vi "AOD Control (host).vi"() -> ()   [LabVIEW 2009]
uses:
  <vilib>/rvi/interface/nirviOpenFPGA/nirviOpenFPGA.xnode
  <vilib>/rvi/interface/nirviReadWriteControl/nirviReadWriteControl.xnode
  <vilib>/rvi/interface/nirviMethod/nirviMethod.xnode
  <vilib>/LabVIEW Targets/FPGA/Rio/nirio_PxiTriggers.ctl
  <vilib>/rvi/interface/nirviCloseFPGA/nirviCloseFPGA.xnode
  C:/Program Files/National Instruments/LabVIEW 2009/resource/objmgr/daqmx.rc
  <vilib>/Utility/error.llb/DialogType.ctl
  <vilib>/DAQmx/write.llb/DAQmx Write (Digital Bool 1Line 1Point).vi
  <vilib>/Analysis/NI_AALBase.lvlib
  <instrlib>/niHWS/nihws.llb/niHWS Write Analog I32.vi
  <instrlib>/niHWS/nihws.llb/niHWS Open File Permissions ID.ctl
  <vilib>/DAQmx/create/channels.llb/DAQmx Create Channel (DO-Digital Output).vi
  <vilib>/DAQmx/read.llb/DAQmx Read (Raw 1D I32).vi
  <instrlib>/niHWS/nihws.llb/niHWS Write Analog I16.vi
  <vilib>/DAQmx/write.llb/DAQmx Write (Analog DBL 1Chan 1Samp).vi
  FPGA Bitfiles/AOD Control.lvproj_PXI-7954R_AOD Control (FPGA)~D2.lvbitx
  AOD Control (FPGA).vi
  AODRef.ctl
  FPGA Bitfiles/AOD Control.lvproj_PXIe-7965R_AOD Control (FPGA)~D2.lvbitx
  <vilib>/FPGA/interface/niFpgaViExecutionMode.ctl
  <vilib>/rvi/errors/niLvFpgaMergeErrorWithErrorCode.vi
  <vilib>/rvi/interface/RandomDataEmulation/nirviRandomDataDMAMethods.vi
  <vilib>/rvi/interface/common/niFpgaNodeNameForErrorReporting.ctl
  <vilib>/rvi/interface/RandomDataEmulation/niFpgaReadControlTemplate.vi
  <vilib>/rvi/interface/RandomDataEmulation/nirviRandomDataRunMethod.vi
  <vilib>/rvi/interface/RandomDataEmulation/niFpgaWriteControlTemplate.vi
  <vilib>/rvi/interface/RandomDataEmulation/nirviRandomDataClose.vi
  <vilib>/userdefined/High Color/nirio_resource_hc.ctl
panel:
  in  "Max":u32=700000
  in  "GridPoints":dbl=5.0
  in  "Power":dbl(slide) min=0.0 max=5.0 step=0.1 scale=0.0..5.0
  out "OutOfRange":bool
  out "Processing":bool
  out "Acquire":bool
  out "FPGA State":T1(ring)
  out "Host State":T2(ring)
  out "Scanning Your Mom":dbl(slide) scale=0.0..1.0
  in  "Tab Control":T3(tab)=enum."Miscellaneous"
  in  "Display Data":bool=TRUE
  in  "ClearPoints":bool
  in  "Scan Settings":T4={"XStart"=-200000000, "XEnd"=200000000, "XNum"=500, "YStart"=-200000000, "YEnd"=200000000, "YNum"=500, "ZStart"=0, "ZEnd"=0, "ZNum"=1}
  in  "Points":i32[][](array[numeric])
  in  "Stop":bool
  in  "Scan":bool
  in  "Volume Scan":bool
  in  "Abort":bool
  in  "Reset":bool
  out "Writing":bool
  in  "SaveStream":bool
  in  "SaveImage":bool
  in  "Path":path
  in  "Scans":i32=5
  in  "ImCh1":bool=TRUE
  in  "Ephys":bool
  in  "Photodiode":bool
  in  "ImCh2":bool
  in  "Throwaway (us)":i32=10
  out "PointArray":cluster{"X":i32, "Y":i32, "Z":i32}[](array[cluster])
  out "StreamInfo":T5
  in  "Downsample":i32=40
  in  "DDS SysClk":i32=100000000
  in  "FPGA Clk":i32=40000000
  in  "ImReadSize":i32=10000
  in  "AcqDivider":i32=20
  out "Acq Freq":dbl format="%#_8g"
  out "Loop Count":i32
  out "PointTime":u32
  out "PMT FIFO Space":u32
  out "ImCh Backlog":u32
  out "FPGA PMT Remaining":u32
  out "PMT Backlog":u32
  out "Command":i16
  in  "P high":u32=10
  in  "P":bool
  out "PMT Read":i32
  out "FPGA Loop Count":i32
  out "Point":cluster{"X":i32, "Y":i32, "Z":i32}
  out "TotalSamples":u32
  out "Written":cluster{"Address":u8, "Value":u32}[](array[cluster]) {"Address" format="%x"; "Value" format="%x"}
  out "PMT Array":i32[](array[numeric])
  out "ImCh Read":i32
  out "Mode":enum16{"Points", "Volume", "Idle"}(ring)
  out "FPGA VI Execution Mode":T6
  out "StackSize":cluster{"nX":u32, "nY":u32, "nZ":u32}
  out "raw out":refnum<queue>
  out "voxel queue":refnum<queue>
  out "NumChans":u32
  out "XPos":i32[](array[numeric])
  out "TRIG0":bool
  out "ExtAcqTrig":bool
  out "TriggerAcq":bool=TRUE
  out "Armed":bool
  out "Bad PMTData":bool
  out "SerialError":bool
  out "Sequencing error":bool
  out "YPos":i32[](array[numeric])
  out "ZPos":i32[](array[numeric])
  out "Point Freq":dbl
  out "SampleCount":u32
  out "AcqDivCount":u32
  out "# pending remove":i32
  out "Processed":i32
  in  "BlankTime (us)":i16=10
  out "BlankSamples":u32
  out "Throwaway Samples":dbl
  out "RepNum":i32
  out "NumReps":i32
  out "NumPoints":i32
  out "PointNum":u32
  out "LaserPowerTask":refnum<k21>
  in  "Execute":bool
  in  "Debug Mode":T7(ring)
  in  "Space":i32
  in  "decimating factor":i32=10
  in  "BaselineRate":dbl=0.01 min=0.0 max=1.0
  in  "RIO Device":T8="RIO0"
  out "ImData":i32[][](array[numeric])
  out "ImCh1 2":T9(plugin-control)
  out "ImCh2 2":T9(plugin-control)
  in  "Section":i32(c297)
  out "Waveform Chart":waveform(dbl)[](graph)
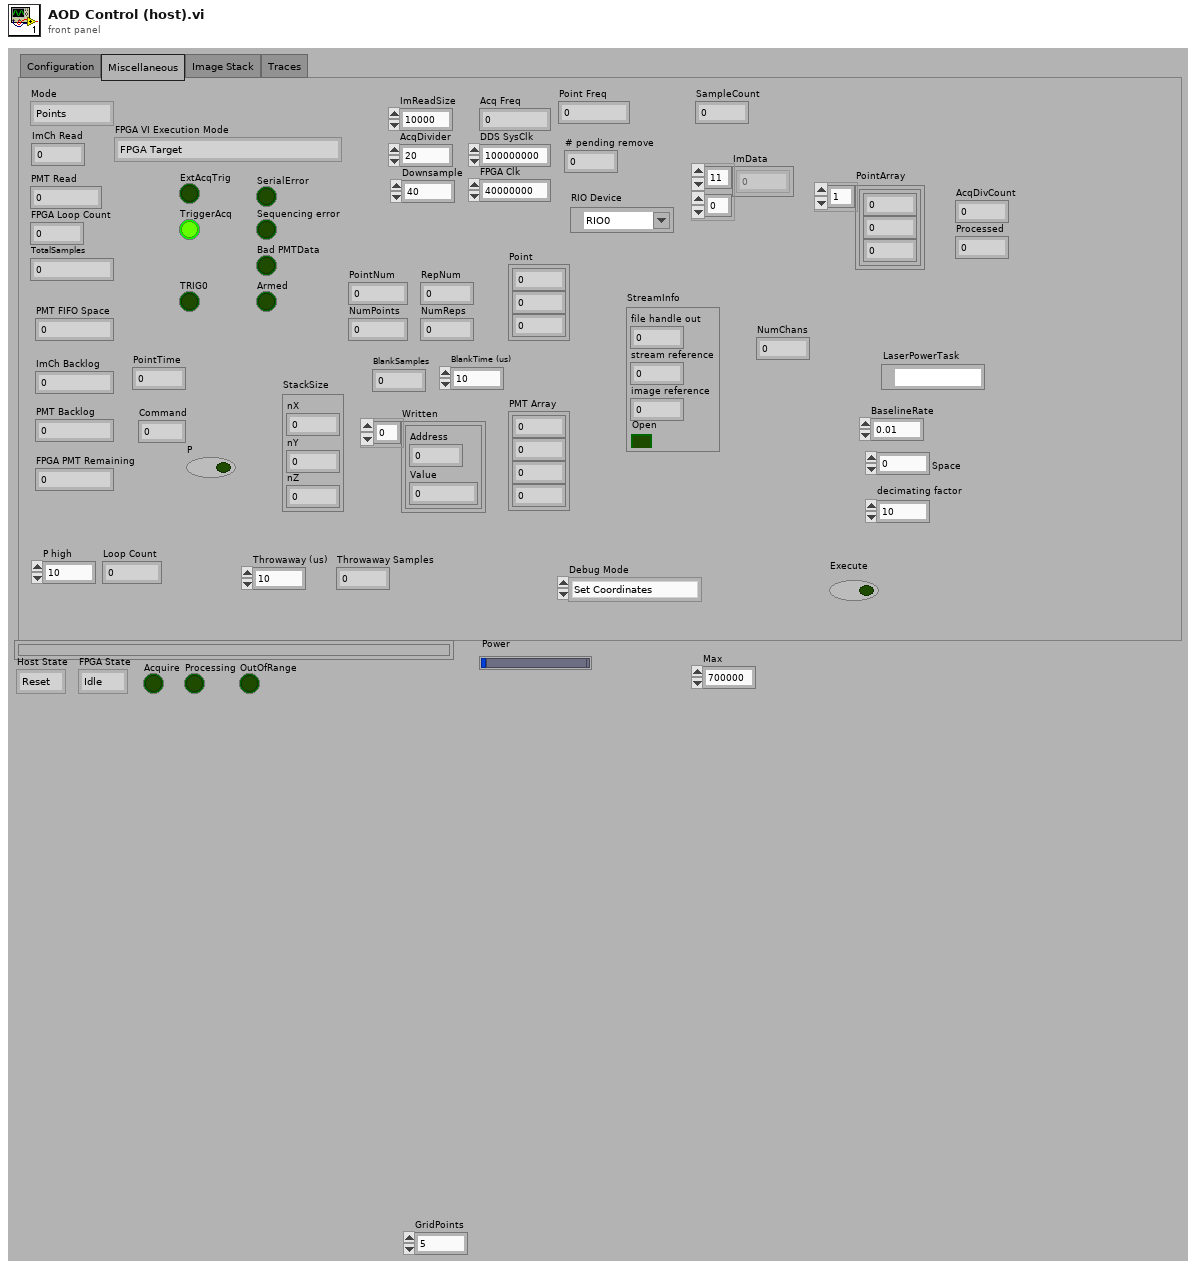
[diagram p1: front panel]
types:
  T1 = enum16{"Idle", "Write Registers", "Receive Points", "Prepare Volume", "Arm Scan", "Scan Points"}
  T2 = enum16{"Reset", "Idle", "Start Acquire", "Acquire", "End Acquire"}
  T3 = enum32{"Configuration", "Miscellaneous", "Image Stack", "Traces"}
  T4 = cluster{"XStart":i32, "XEnd":i32, "XNum":i32, "YStart":i32, "YEnd":i32, "YNum":i32, "ZStart":i32, "ZEnd":i32, "ZNum":i32}
  T5 = cluster{"file handle out":u32, "stream reference":u32, "image reference":u32, "Open":bool}
  T6 = typedef "niFpgaViExecutionMode.ctl" = enum16{"FPGA Target", "Development Computer with Simulated I/O", "Development Computer with Real I/O"}
  T7 = enum16{"Set Coordinates", "Toggle Axis", "Sweep Settings"}
  T8 = typedef "nirio_resource_hc.ctl" = tag
  T9 = typedef "IMAQ Image.ctl" = refnum<image>
  T10 = typedef "AODRef.ctl" = refnum<k20>
  T11 = typedef "nirio_PxiTriggers.ctl" = u16
  T12 = typedef "niFpgaNodeNameForErrorReporting.ctl" = enum16{"Open FPGA VI Reference", "Read/Write Control", "Invoke Method: Abort", "Invoke Method: Acknowledge IRQ", "Invoke Method: Download", "Invoke Method: FIFO.Configure", "Invoke Method: FIFO.Read", "Invoke Method: FIFO.Start", "Invoke Method: FIFO.Stop", "Invoke Method: FIFO.Write", "Invoke Method: Reset", "Invoke Method: Run", "Invoke Method: Wait on IRQ", "Close FPGA VI Reference"}
  T13 = typedef "niHWS Open File Permissions ID.ctl" = enum32{"Read Only", "Read/Write Existing", "Read/Write/Create New", "Read/Write/Create New Always"}
  T14 = typedef "Image Type" = u32
  T15 = typedef "DialogType.ctl" = u16
  T16 = cluster{"Global Rectangle":i32[], "Contours":cluster{"Contour Type":u32, "ROI Type":u32, "Points":i32[]}[]}
  T17 = cluster{"Global Rectangle":i32[], "Contours":cluster{"Contour Type":u32, "ROI Type":u32, "Points":i32[]}[]}[]
  T18 = cluster{"Contour Type":u32, "ROI Type":u32, "Points":i32[]}[]
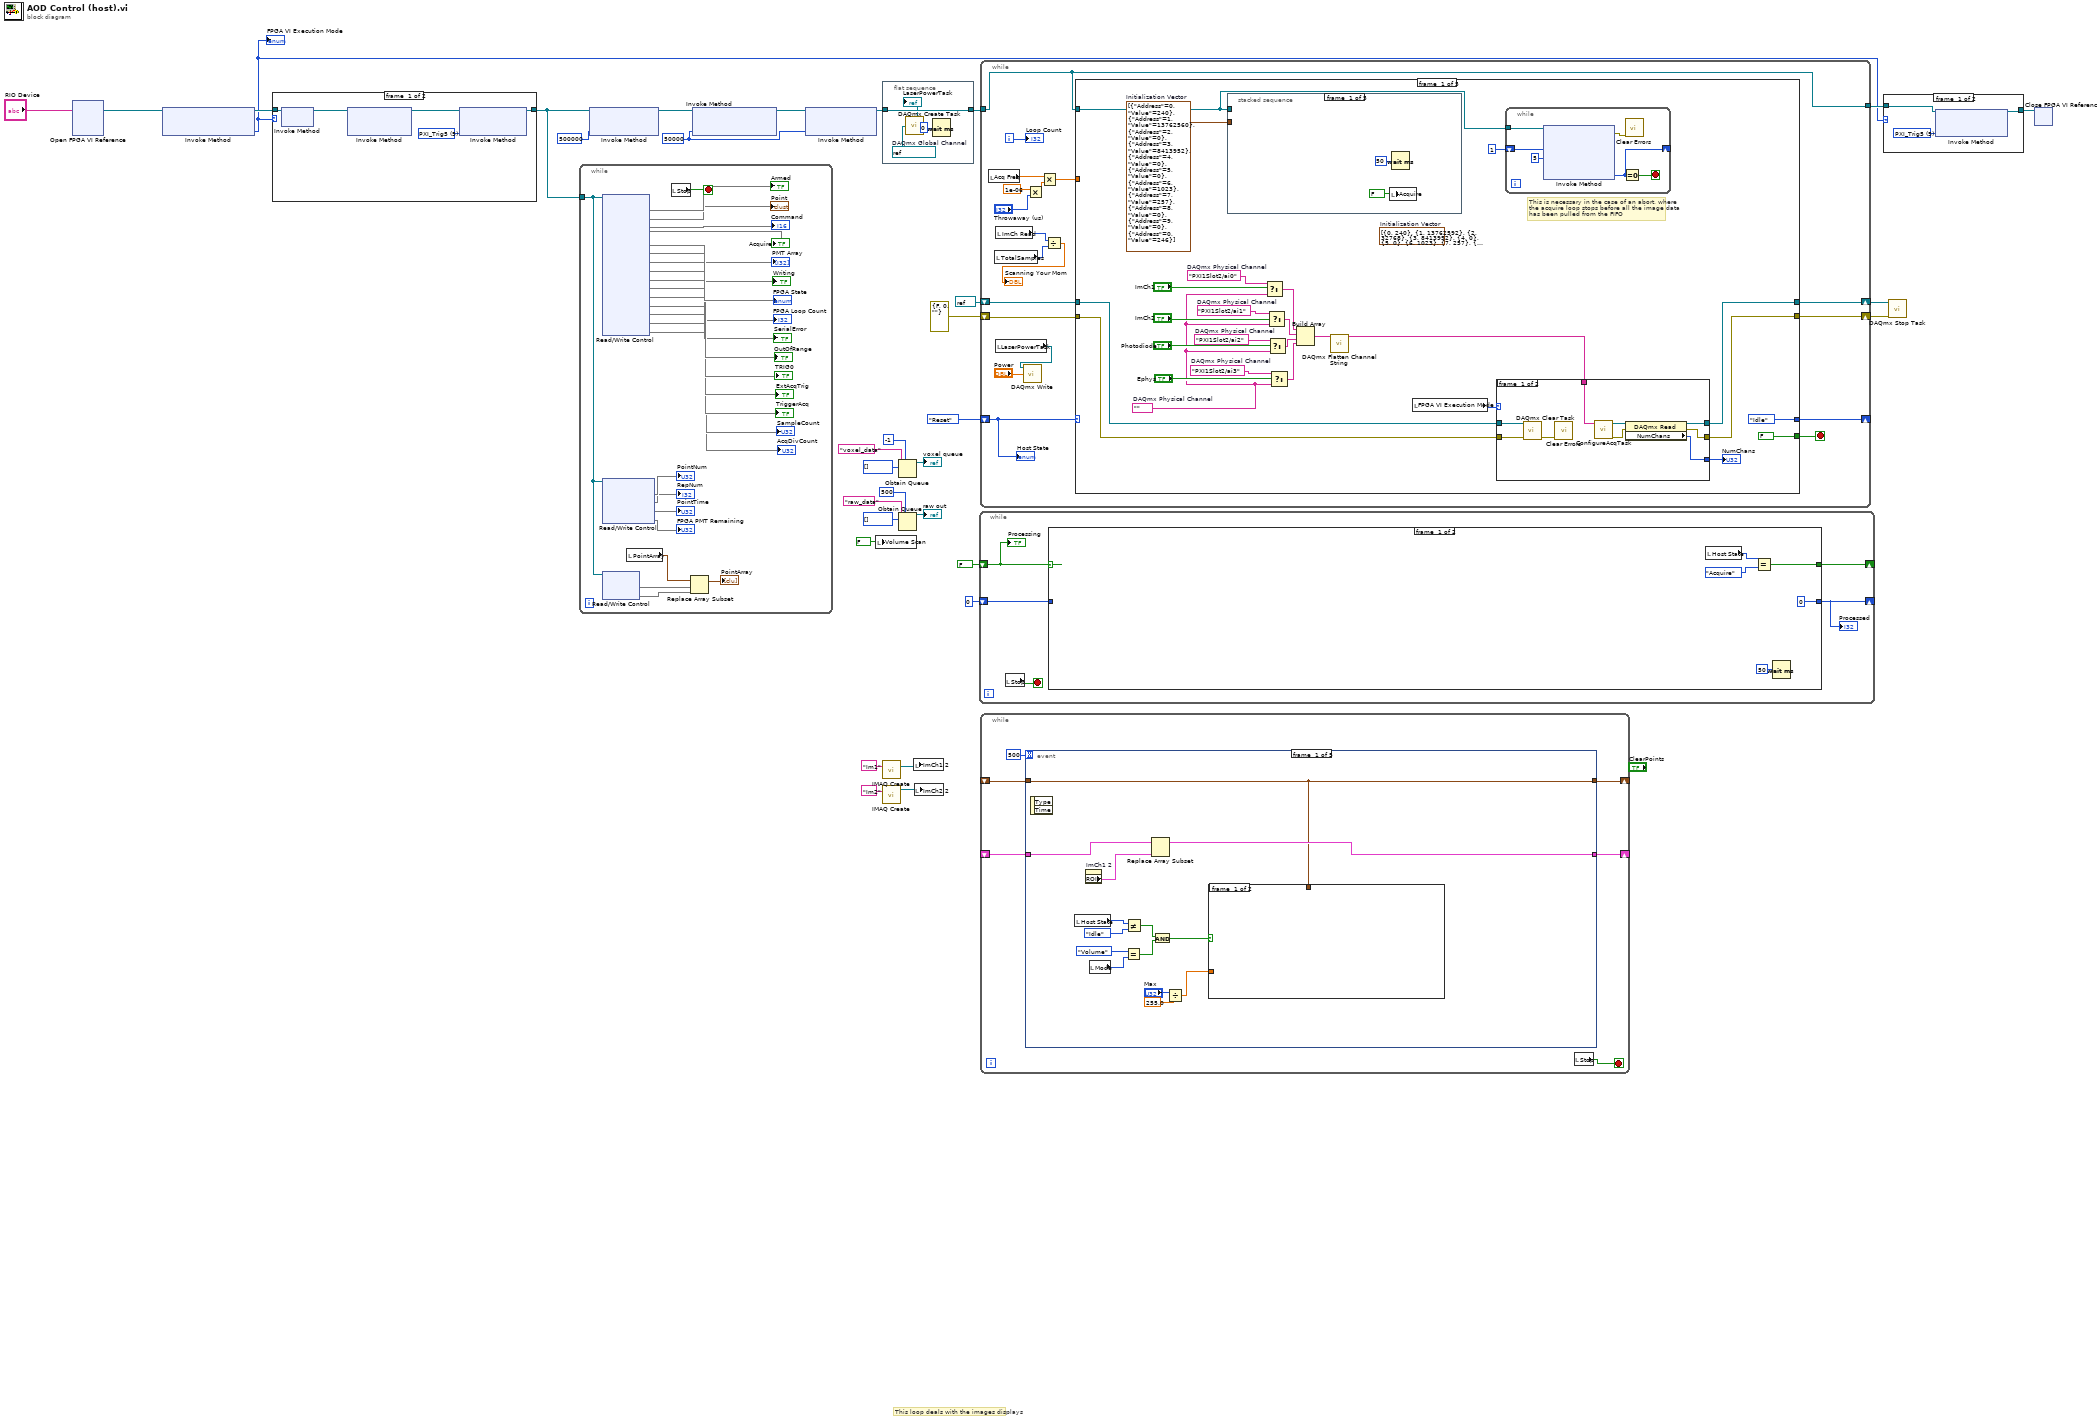
[diagram p0: block diagram]
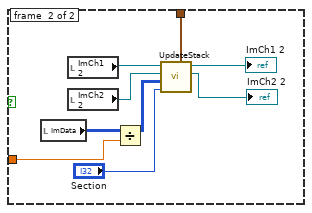
[diagram p2: hidden frame]
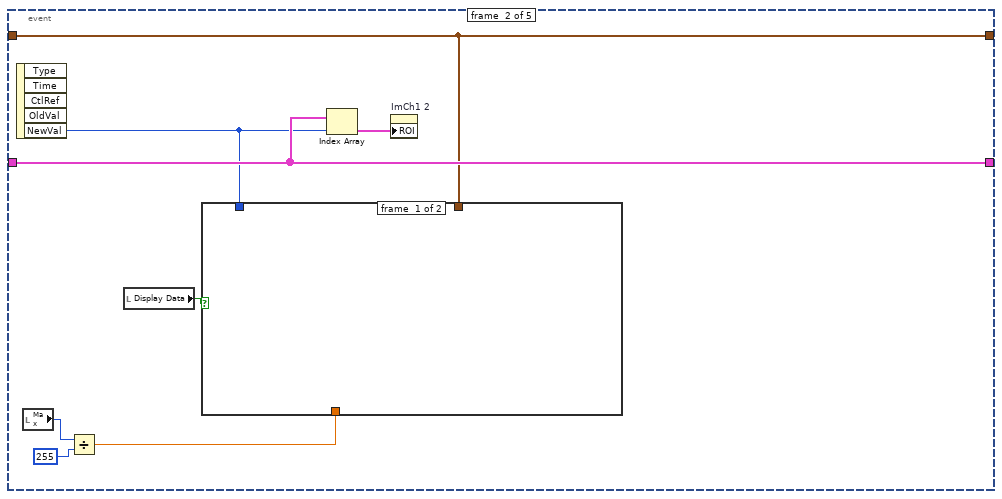
[diagram p3: hidden frame]
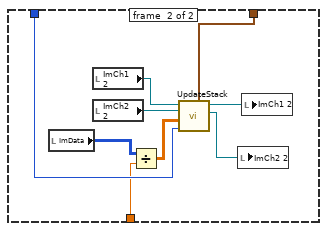
[diagram p4: hidden frame]
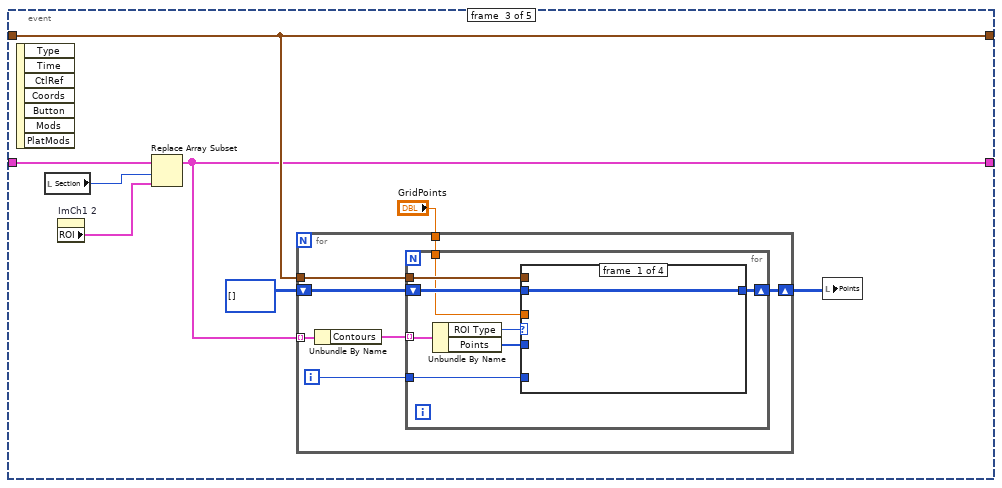
[diagram p5: hidden frame]
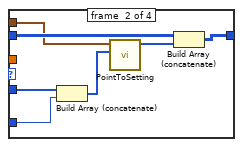
[diagram p6: hidden frame]
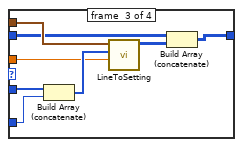
[diagram p7: hidden frame]
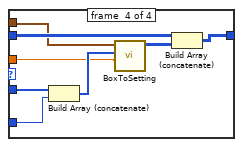
[diagram p8: hidden frame]
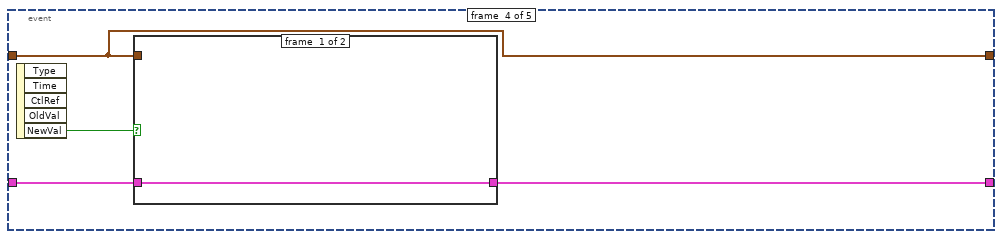
[diagram p9: hidden frame]
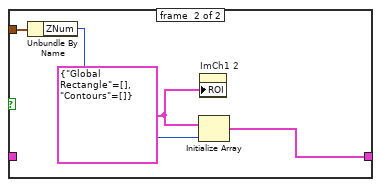
[diagram p10: hidden frame]
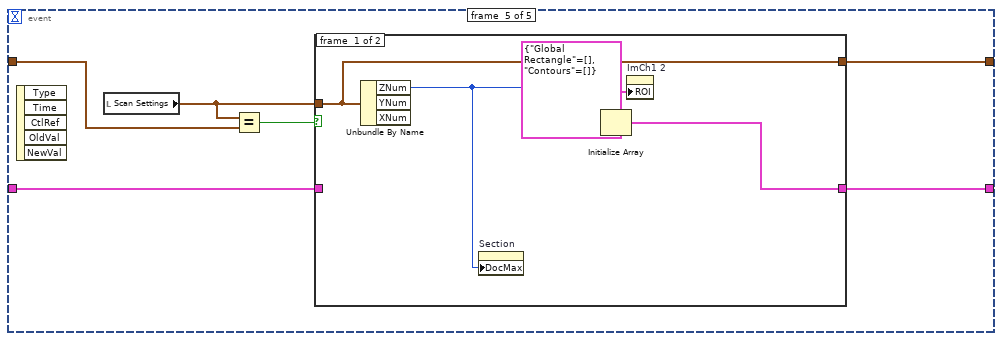
[diagram p11: hidden frame]
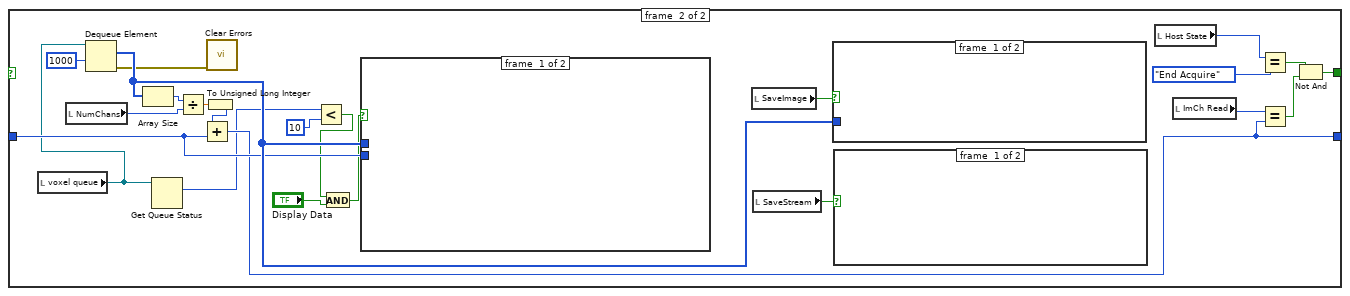
[diagram p13: hidden frame]
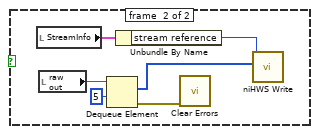
[diagram p14: hidden frame]
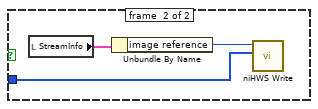
[diagram p15: hidden frame]
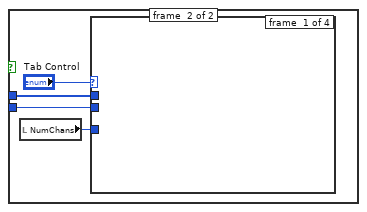
[diagram p16: hidden frame]
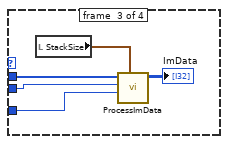
[diagram p18: hidden frame]
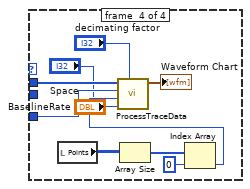
[diagram p19: hidden frame]
diagram:
  w29 = u32 50000 ("Depth")
  # "This loop deals with the images displays"
  n1 = xnode "Open FPGA VI Reference"("resource name"="RIO Device") -> ("FPGA VI Reference Out"=w33:T10)  [unwired: 1 in, 1 out]
  n2 = xnode "Invoke Method"("FPGA VI Reference In"=w33) -> ("FPGA VI Reference Out"=w20:T10, "FPGA VI Execution Mode"=w19:T6)  [unwired: 1 in, 1 out]
  "FPGA VI Execution Mode" <- w19
  n3 = case shown="\"FPGA Target\", Default" w19 {
    tunnel: [w34 w59] -> w7
    tunnel: w20 -> [w38 w59]
    frame #0 {
      w36 = T11 5 items=["PXI_Trig0", "PXI_Trig1", "PXI_Trig2", "PXI_Trig3", "PXI_Trig4", "PXI_Trig5", "PXI_Trig6", "PXI_Trig7"] ("Trigger")
      n4 = xnode "Invoke Method"("FPGA VI Reference In"=w38) -> ("FPGA VI Reference Out"=w37:T10)  [unwired: 1 in, 1 out]
      n5 = xnode "Invoke Method"("FPGA VI Reference In"=w37) -> ("FPGA VI Reference Out"=w35:T10)  [unwired: 2 in, 1 out]
      n6 = xnode "Invoke Method"("FPGA VI Reference In"=w35, "Trigger"=w36) -> ("FPGA VI Reference Out"=w34:T10)  [unwired: 1 in, 1 out]
    }
    frame #1 {
    }
  }
  n7 = while {
    tunnel: w7 -> [w66]
    stop <- w84 stop-if-true
    n8 = xnode "Read/Write Control"("FPGA VI Reference In"=w66) -> ("Armed"=→"Armed", "Point"=→"Point", "Command"=→"Command", "Acquire"=→"Acquire", "PMT Array"=→"PMT Array":void[], "Writing"=→"Writing", "State"=→"FPGA State", "Count"=→"FPGA Loop Count", "SerialError"=→"SerialError", "OutOfRange"=→"OutOfRange", "TRIG0"=→"TRIG0", "ExtAcqTrig"=→"ExtAcqTrig", "TriggerAcq"=→"TriggerAcq", "SampleCount"=→"SampleCount", "AcqDivCount"=→"AcqDivCount")  [unwired: 1 in, 2 out]
    n9 = xnode "Read/Write Control"("FPGA VI Reference In"=w66) -> ("PointNum"=→"PointNum", "RepNum"=→"RepNum", "PointTime"=→"PointTime", "PMT Remaining"=→"FPGA PMT Remaining")  [unwired: 1 in, 2 out]
    n10 = xnode "Read/Write Control"("FPGA VI Reference In"=w66) -> ("PointNum"=w63, "Point"=w62)  [unwired: 1 in, 2 out]
    n11 = local read "PointArray"() -> (w65:cluster{"X":i32, "Y":i32, "Z":i32}[])
    n12 = local read "Stop"() -> (w84:bool)
    n13 = Replace Array Subset(array=w65, new element=w62, index=w63) -> (→"PointArray":cluster{"X":i32, "Y":i32, "Z":i32}[])
  }
  n14 = xnode "Invoke Method"("FPGA VI Reference In"=w7, "Depth"=u32 500000) -> ("FPGA VI Reference Out"=w22:T10)  [unwired: 1 in, 1 out]
  n15 = xnode "Invoke Method"("FPGA VI Reference In"=w22, "Depth"=w29) -> ("FPGA VI Reference Out"=w21:T10)  [unwired: 1 in, 1 out]
  n16 = xnode "Invoke Method"("FPGA VI Reference In"=w21, "Depth"=w29) -> ("FPGA VI Reference Out"=w24:T10)  [unwired: 1 in, 1 out]
  n17 = local write "Volume Scan"(FALSE ("Volume Scan")) -> ()
  n18 = call "IMAQ Create"("Image Name"="Im1") -> ("New Image"=w2:T9)  [unwired: 4 in, 1 out]
  n19 = call "IMAQ Create"("Image Name"="Im2") -> ("New Image"=w1:T9)  [unwired: 4 in, 1 out]
  n20 = flat-sequence {
    tunnel: [w115] -> w23
    tunnel: w24 -> [w115]
    frame #0 {
      w112 = refnum<k21> "AOD Gain"  # DAQmx Global Channel
      n21 = call <vilib>:"DAQmx Create Task.vi"("global virtual channels"=w112) -> ("task out"=→"LaserPowerTask":refnum<k21>)  [unwired: 4 in, 10 out]
      n22 = Wait (ms)(milliseconds to wait=u32 0) -> ()  [unwired: 1 out]
    }
  }
  n23 = Obtain Queue(max queue size (-1, unlimited)=-1, name (unnamed)="voxel_data", element data type=u32[] [] ("data")) -> (queue out=→"voxel queue":refnum<queue>)  [unwired: 2 in, 2 out]
  n24 = Obtain Queue(max queue size (-1, unlimited)=500, name (unnamed)="raw_data", element data type=u32[] [] ("data")) -> (queue out=→"raw out":refnum<queue>)  [unwired: 2 in, 2 out]
  n25 = local write "ImCh1 2"(w2) -> ()
  n26 = local write "ImCh2 2"(w1) -> ()
  n27 = while {
    shift-right: [w116] -> _
    shift-left: 0 -> [w119]
    shift-right: [w118] -> _
    shift-left: FALSE -> [w117]
    stop <- w120 stop-if-true
    n28 = local read "Stop"() -> (w120:bool)
    n29 = case shown="True" w117 {
      tunnel: w119 -> [_ w142]
      tunnel: [0 w138] -> w116
      tunnel: [w121 w137] -> w118
      frame #0 {
        n30 = local read "Host State"() -> (w122:T2)
        n31 = Equal?(x=w122, y=T2."Acquire") -> (x = y?=w121:bool)
        n32 = Wait (ms)(milliseconds to wait=u32 50) -> ()  [unwired: 1 out]
      }
      frame #1 {
        n33 = local read "voxel queue"() -> (w133:refnum<queue>)
        n34 = local read "NumChans"() -> (w131:u32)
        n35 = Dequeue Element(queue=w133, timeout in ms (-1)=1000) -> (element=w146:u32[], error out=w143:errorcluster)  [unwired: 1 in, 2 out]
        n36 = Array Size(array=w146) -> (size(s)=w132:i32)
        n37 = Get Queue Status(queue=w133) -> (# pending remove=w134:i32)  [unwired: 2 in, 7 out]
        n38 = Divide(x=w132, y=w131) -> (x/y=w130:dbl)
        n39 = To Unsigned Long Integer(number=w130) -> (unsigned 32bit integer=w129:u32)
        n40 = Add(x=w129, y=w142) -> (x+y=w138:u32)
        n41 = call <vilib>:"Clear Errors.vi"("error in (no error)"=w143) -> ()  [unwired: 6 in, 1 out]
        n42 = Less?(x=w134, y=10) -> (x < y?=w127:bool)
        n43 = And(x=w127, y="Display Data") -> (x .and. y?=w126:bool)
        n44 = case shown="True" w126 {
          tunnel: w146 -> [_ w160]
          tunnel: w142 -> [_ w159]
          frame #0 {
          }
          frame #1 {
            n45 = local read "NumChans"() -> (w158:u32)
            n46 = case shown="\"Image Stack\"" "Tab Control" {
              tunnel: w160 -> [_ _ w166 w176]
              tunnel: w159 -> [_ _ w165 _]
              tunnel: w158 -> [_ _ w163 w175]
              frame #0 {
              }
              frame #1 {
              }
              frame #2 {
                n47 = local read "StackSize"() -> (w164:cluster{"nX":u32, "nY":u32, "nZ":u32})
                n48 = call "ProcessImData.vi"("StackSize"=w164, "NumChans"=w163, "StartingNum"=w165, "Data"=w166) -> ("output array"=→"ImData":i32[][])  [unwired: 7 in]
              }
              frame #3 {
                n49 = local read "Points"() -> (w174:i32[][])
                n50 = Array Size(array=w174) -> (size(s)=w173:i32[])
                n51 = Index Array(array=w173, index=0) -> (element=w171:i32)
                n52 = call "ProcessTraceData.vi"("BaselineRate"="BaselineRate", "decimating factor"="decimating factor", "Space"="Space", "NumPoints"=w171, "NumChans"=w175, "Data"=w176) -> ("Waveforms"=→"Waveform Chart":waveform(dbl)[])  [unwired: 5 in]
              }
            }
          }
        }
        n53 = local read "SaveImage"() -> (w147:bool)
        n54 = local read "SaveStream"() -> (w145:bool)
        n55 = case shown="True" w147 {
          tunnel: w146 -> [_ w155]
          frame #0 {
          }
          frame #1 {
            n56 = local read "StreamInfo"() -> (w157:T5)
            n57 = Unbundle By Name(w157) -> ("image reference"=w156:u32)
            n58 = call-poly <instrlib>:"niHWS Write.vi"("data"=w155, "waveform reference in"=w156) -> ()  [unwired: 8 in, 2 out]
          }
        }
        n59 = case shown="True" w145 {
          frame #0 {
          }
          frame #1 {
            n60 = local read "StreamInfo"() -> (w154:T5)
            n61 = local read "raw out"() -> (w152:refnum<queue>)
            n62 = Dequeue Element(queue=w152, timeout in ms (-1)=5) -> (element=w151:u32[], error out=w149:errorcluster)  [unwired: 1 in, 2 out]
            n63 = Unbundle By Name(w154) -> ("stream reference"=w153:u32)
            n64 = call <vilib>:"Clear Errors.vi"("error in (no error)"=w149) -> ()  [unwired: 6 in, 1 out]
            n65 = call-poly <instrlib>:"niHWS Write.vi"("data"=w151, "waveform reference in"=w153) -> ()  [unwired: 8 in, 2 out]
          }
        }
        n66 = local read "Host State"() -> (w140:T2)
        n67 = local read "ImCh Read"() -> (w139:i32)
        n68 = Equal?(x=w140, y=T2."End Acquire") -> (x = y?=w136:bool)
        n69 = Equal?(x=w139, y=w138) -> (x = y?=w135:bool)
        n70 = Not And(1:w135, 2:w136) -> (0:w137:bool)
      }
    }
    "Processed" <- w116
    "Processing" <- w117
  }
  n71 = while {
    tunnel: w23 -> [w187]
    tunnel: [w187] -> w30
    shift-right: [w189] -> _
    shift-left: T2."Reset" -> [w190]
    shift-right: [w194] -> w28
    shift-left: refnum<k21> refnum ("task out") -> [w192]
    shift-right: [w193] -> w27
    shift-left: errorcluster {"status"=FALSE, "code"=0, "source"=""} ("error out") -> [w191]
    i -> [w195]
    stop <- w188 stop-if-true
    n72 = local read "Acq Freq"() -> (w180:dbl)
    n73 = local read "TotalSamples"() -> (w185:u32)
    n74 = local read "LaserPowerTask"() -> (w178:refnum<k21>)
    n75 = local read "ImCh Read"() -> (w186:i32)
    n76 = call-poly <vilib>:"DAQmx Write.vi"("task/channels in"=w178, "data"="Power") -> ()  [unwired: 11 in, 3 out]
    n77 = Multiply(x=1e-06, y="Throwaway (us)") -> (x*y=w181:dbl)
    n78 = Multiply(x=w180, y=w181) -> (x*y=w179:dbl)
    n79 = Divide(x=w186, y=w185) -> (x/y=→"Scanning Your Mom":dbl)
    n80 = case shown="\"Idle\"" w190 {
      selector: w190 -> [_ w453 _ _ _]
      tunnel: w191 -> [w219 w452 w506 w853 w1004]
      tunnel: w192 -> [w218 w427 w507 w854 w998]
      tunnel: [w215 w427 w504 w867 w998] -> w194
      tunnel: [w216 w452 w505 w855 w999] -> w193
      tunnel: [T2."Idle" w441 T2."Acquire" w866 w997] -> w189
      tunnel: w187 -> [w212 w442 w508 w839 w1001]
      tunnel: [FALSE ("Stop") "Stop" FALSE ("Stop") FALSE ("Stop") FALSE ("Stop")] -> w188
      tunnel: w179 -> [_ _ _ w828 _]
      frame #0 {
        w196 = tag ""  # DAQmx Physical Channel
        w197 = tag "PXI1Slot2/ai3"  # DAQmx Physical Channel
        w198 = tag "PXI1Slot2/ai2"  # DAQmx Physical Channel
        w199 = tag "PXI1Slot2/ai1"  # DAQmx Physical Channel
        w200 = tag "PXI1Slot2/ai0"  # DAQmx Physical Channel
        w217 = cluster{"Address":u8, "Value":u32}[] [{"Address"=0, "Value"=240}, {"Address"=1, "Value"=13762560}, {"Address"=2, "Value"=0}, {"Address"=3, "Value"=8413952}, {"Address"=4, "Value"=0}, {"Address"=5, "Value"=0}, {"Address"=6, "Value"=1023}, {"Address"=7, "Value"=257}, {"Address"=8, "Value"=0}, {"Address"=9, "Value"=0}, {"Address"=0, "Value"=246}]  # Initialization Vector
        (unwired) cluster{"Address":u8, "Value":u32}[] [{"Address"=0, "Value"=240}, {"Address"=1, "Value"=13762592}, {"Address"=2, "Value"=32768}, {"Address"=3, "Value"=8413952}, {"Address"=4, "Value"=0}, {"Address"=5, "Value"=0}, {"Address"=6, "Value"=1023}, {"Address"=7, "Value"=257}, {"Address"=8, "Value"=21}, {"Address"=4, "Value"=858993459}]  # Initialization Vector
        # "This is necessary in the case of an abort, where \nthe acquire loop stops before all the image data\nhas been pulled from the FIFO"
        n81 = stacked-sequence {
          tunnel: w212 -> [_ w258 w281 w334 w352]
          tunnel: w217 -> [_ _ w278 _ _]
          frame #0 {
            n82 = local write "Acquire"(FALSE ("Acquire")) -> ()
            n83 = Wait (ms)(milliseconds to wait=u32 50) -> ()  [unwired: 1 out]
          }
          frame #1 {
            n84 = xnode "Read/Write Control"("FPGA VI Reference In"=w258, "Abort"=FALSE, "Reset"=TRUE) -> ()  [unwired: 1 in, 2 out]
            n85 = Wait (ms)(milliseconds to wait=u32 10) -> ()  [unwired: 1 out]
          }
          frame #2 {
            n86 = Wait (ms)(milliseconds to wait=u32 500) -> ()  [unwired: 1 out]
            n87 = Array Size(array=w278) -> (size(s)=w284:i32)
            n88 = xnode "Read/Write Control"("FPGA VI Reference In"=w281, "Register Writes"=w278, "Number Registers"=w284, "Write Register"=FALSE, "WriteSize"=enum16{"1", "2", "4"}."1", "SclkDivider"=u32 4 ("ClockPause"), "stop"=FALSE, "Downsample"=40, "Reset"=FALSE, "PMT Timeout"=20000000) -> ()  [unwired: 1 in, 2 out]
          }
          frame #3 {
            n89 = xnode "Read/Write Control"("FPGA VI Reference In"=w334, "Write Register"=TRUE) -> ()  [unwired: 1 in, 2 out]
            n90 = Wait (ms)(milliseconds to wait=u32 10) -> ()  [unwired: 1 out]
          }
          frame #4 {
            n91 = xnode "Read/Write Control"("FPGA VI Reference In"=w352, "Write Register"=FALSE, "WriteSize"=enum16{"1", "2", "4"}."4", "SclkDivider"=u32 2 ("ClockPause"), "Pause"=u32 4, "UpdateIO time"=u32 4) -> ()  [unwired: 1 in, 2 out]
          }
        }
        n92 = Select(t=w200, s="ImCh1", f=w196) -> (s? t:f=w203:tag)
        n93 = Select(t=w199, s="ImCh2", f=w196) -> (s? t:f=w202:tag)
        n94 = Select(t=w198, s="Photodiode", f=w196) -> (s? t:f=w206:tag)
        n95 = Select(t=w197, s="Ephys", f=w196) -> (s? t:f=w208:tag)
        n96 = Build Array(w203, w202, w206, w208) -> (w210:tag[])
        n97 = call <vilib>:"DAQmx Flatten Channel String.vi"("names in"=w210) -> ("names out"=w201:string)  [unwired: 13 in, 1 out]
        n98 = local read "FPGA VI Execution Mode"() -> (w214:T6)
        n99 = case shown="\"FPGA Target\", Default" w214 {
          tunnel: w219 -> [w251 w253]
          tunnel: w218 -> [w250 w254]
          tunnel: [w245 w253] -> w216
          tunnel: [w246 w254] -> w215
          tunnel: [w244 u32 1 ("NumChans")] -> w213
          tunnel: w201 -> [w243 _]
          frame #0 {
            n100 = call <vilib>:"DAQmx Clear Task.vi"("task in"=w250, "error in"=w251) -> ("error out"=w249:errorcluster)  [unwired: 13 in]
            n101 = call <vilib>:"Clear Errors.vi"("error in (no error)"=w249) -> ()  [unwired: 6 in, 1 out]
            n102 = call "ConfigureAcqTask.vi"("AcqCh"=w243) -> ("error out"=w247:errorcluster, "task out"=w248:refnum<k21>)  [unwired: 9 in]
            n103 = property class="DAQmx Read"(reference=w248, error in=w247) -> (reference out=w246:refnum<k21>, error out=w245:errorcluster, "NumChans"=w244:u32)
          }
          frame #1 {
          }
        }
        "NumChans" <- w213
        n104 = while {
          tunnel: w212 -> [w227]
          shift-right: [w222] -> _
          shift-left: u32 1 ("Number of Elements") -> [w223]
          stop <- w226 stop-if-true
          n105 = xnode "Invoke Method"("FPGA VI Reference In"=w227, "Number of Elements"=w223, "Timeout (ms)"=5) -> ("error out"=w224:errorcluster, "Elements Remaining"=w222:u32)  [unwired: 1 in, 2 out]
          n106 = Equal To 0?(x=w222) -> (x = 0?=w226:bool)
          n107 = call <vilib>:"Clear Errors.vi"("error in (no error)"=w224) -> ()  [unwired: 6 in, 1 out]
        }
      }
      frame #1 {
        w385 = u32 858993459 ("LP Center Frequency")
        w418 = FALSE
        w414 = T2."Start Acquire"
        n108 = local read "NumChans"() -> (w412:u32)
        n109 = local read "Scans"() -> (w419:i32)
        n110 = local read "voxel queue"() -> (w408:refnum<queue>)
        n111 = local read "Volume Scan"() -> (w421:bool)
        n112 = xnode "Read/Write Control"("FPGA VI Reference In"=w442, "stop"="Stop", "Channels"=w412, "AcqDivider"="AcqDivider", "NumReps"=w419, "TriggerAcq"=w418, "ExtAcqTrig"=w418, "HP Center Frequency"=w385, "LP Center Frequency"=w385) -> ("FPGA VI Reference Out"=w447:T10, "Sequencing error"=→"Sequencing error")  [unwired: 1 in, 1 out]
        n113 = local read "Points"() -> (w405:i32[][])
        n114 = Get Queue Status(queue=w408) -> (# pending remove=→"# pending remove":i32)  [unwired: 2 in, 7 out]
        n115 = Array Size(array=w405) -> (size(s)=w404:i32[])
        n116 = Divide(x="FPGA Clk", y="AcqDivider") -> (x/y=w398:dbl)
        "Acq Freq" <- w398
        n117 = Index Array(array=w404, index=0) -> (element=w402:i32)
        n118 = feedback #1() -> (w423:bool)  [unwired: 1 in]
        n119 = Not(x=w423) -> (.not. x?=w422:bool)
        n120 = Greater Than 0?(x=w402) -> (x > 0?=w400:bool)
        n121 = Divide(x="DDS SysClk", y=w398) -> (x/y=w434:dbl)
        n122 = And(x=w421, y=w422) -> (x .and. y?=w420:bool)
        n123 = And(x="Scan", y=w400) -> (x .and. y?=w399:bool)
        n124 = Multiply(x="Downsample", y=w434) -> (x*y=w436:dbl)
        n125 = feedback #2() -> (w431:bool)  [unwired: 1 in]
        n126 = Not(x=w431) -> (.not. x?=w432:bool)
        n127 = Round Toward +Infinity(x=w436) -> (ceil(x): smallest int >= x=w435:dbl)
        n128 = Divide(x=w398, y="Downsample") -> (x/y=→"Point Freq":dbl)
        n129 = Multiply(x="BlankTime (us)", y=1e-06) -> (x*y=w397:dbl)
        n130 = To Unsigned Long Integer(number=w435) -> (unsigned 32bit integer=w428:u32)
        n131 = Select(t=w414, s=w420, f=w453) -> (s? t:f=w415:T2)
        n132 = Multiply(x=w397, y=w398) -> (x*y=w394:dbl)
        n133 = And(x=w399, y=w432) -> (x .and. y?=w416:bool)
        n134 = To Unsigned Long Integer(number=w394) -> (unsigned 32bit integer=w393:u32)
        "BlankSamples" <- w393
        n135 = xnode "Read/Write Control"("FPGA VI Reference In"=w447, "Volume Scan"="Volume Scan", "Scan Settings"="Scan Settings", "P"="P", "Downsample"="Downsample", "UpdatesPerPoint"=w428, "P high"="P high", "BlankSamples"=w393) -> ("FPGA VI Reference Out"=w411:T10, "Written"=→"Written":void[], "Bad PMTData"=→"Bad PMTData")  [unwired: 1 in, 2 out]
        n136 = Select(t=w414, s=w416, f=w415) -> (s? t:f=w413:T2)
        n137 = case shown="True" w416 {
          tunnel: w411 -> [_ w459]
          frame #0 {
          }
          frame #1 {
            n138 = call "ScanPoints (host).vi"(7:w459, "Points"="Scans", "FPGA VI Reference Out"="Points") -> ()  [unwired: 9 in]
          }
        }
        n139 = feedback #3() -> (w439:bool)  [unwired: 1 in]
        n140 = Not(x=w439) -> (.not. x?=w438:bool)
        n141 = And(x=w438, y="Reset") -> (x .and. y?=w437:bool)
        n142 = Select(t=T2."Reset", s=w437, f=w413) -> (s? t:f=w441:T2)
        n143 = local read "ImCh Backlog"() -> (w429:u32)
        n144 = xnode "Invoke Method"("FPGA VI Reference In"=w411, "Number of Elements"=w429, "Timeout (ms)"=1) -> ("FPGA VI Reference Out"=w387:T10, "error out"=w430:errorcluster)  [unwired: 1 in, 2 out]
        n145 = feedback #4(TRUE ("Sweep")) -> (w391:bool)
        n146 = Not(x=w391) -> (.not. x?=w390:bool)
        n147 = Wait (ms)(milliseconds to wait=u32 10) -> ()  [unwired: 1 out]
        n148 = And(x=w390, y="Execute") -> (x .and. y?=w388:bool)
        n149 = case shown="True" w388 {
          tunnel: w387 -> [_ w454]
          tunnel: "Debug Mode" -> [_ w455]
          frame #0 {
          }
          frame #1 {
            n150 = case shown="\"Set Coordinates\"" w455 {
              tunnel: w454 -> [_ w456 w457 w458]
              frame #0 {
              }
              frame #1 {
                n151 = call "SetCoordinates.vi"("FPGA VI Reference Out"=w456) -> ()  [unwired: 11 in]
              }
              frame #2 {
                n152 = call "SweepSettings.vi"("FPGA VI Reference Out"=w457) -> ()  [unwired: 11 in]
              }
              frame #3 {
                n153 = call "ToggleAxis.vi"("FPGA VI Reference Out"=w458) -> ()  [unwired: 11 in]
              }
            }
          }
        }
        n154 = call <vilib>:"Clear Errors.vi"("error in (no error)"=w430) -> ()  [unwired: 6 in, 1 out]
      }
      frame #2 {
        n155 = stacked-sequence {
          tunnel: w508 -> [w515 _ w687]
          tunnel: w507 -> [_ _ w686]
          tunnel: w506 -> [_ _ w685]
          tunnel: [_ _ w684] -> w505
          tunnel: [_ _ w683] -> w504
          frame #0 {
            w516 = 0 ("PMT Read")
            w512 = FALSE ("Volume Scan")
            n156 = local read "voxel queue"() -> (w514:refnum<queue>)
            n157 = local read "raw out"() -> (w513:refnum<queue>)
            n158 = xnode "Read/Write Control"("FPGA VI Reference In"=w515) -> ("FPGA VI Reference Out"=w520:T10, "NumPoints"=→"NumPoints", "NumReps"=→"NumReps", "Mode"=w521)  [unwired: 1 in, 1 out]
            "Mode" <- w521
            n159 = local write "Volume Scan"(w512) -> ()
            n160 = local write "Scan"(w512) -> ()
            n161 = local write "PMT Read"(w516) -> ()
            n162 = local write "ImCh Read"(w516) -> ()
            n163 = Flush Queue(queue=w514) -> ()  [unwired: 1 in, 3 out]
            n164 = Flush Queue(queue=w513) -> ()  [unwired: 1 in, 3 out]
            n165 = case shown="\"Volume\"" w521 {
              tunnel: w520 -> [_ w539]
              tunnel: [w530 w538] -> w523
              tunnel: [w526 w536] -> w524
              tunnel: [w528 w534] -> w517
              tunnel: [w526 w537] -> w511
              frame #0 {
                w526 = 0
                n166 = local read "Points"() -> (w533:i32[][])
                n167 = Array Size(array=w533) -> (size(s)=w532:i32[])
                n168 = local write "Tab Control"(T3."Traces" ("Tab Control")) -> ()
                n169 = Index Array(array=w532, index=0) -> (element=w530:i32)
                n170 = local read "Scans"() -> (w529:i32)
                n171 = Multiply(x=w530, y=w529) -> (x*y=w528:i32)
              }
              frame #1 {
                n172 = stacked-sequence {
                  tunnel: w539 -> [w543 w564 w590]
                  frame #0 {
                    n173 = xnode "Read/Write Control"("FPGA VI Reference In"=w543) -> ("Scan Settings.XEnd"=w548, "Scan Settings.XStart"=w544, "Scan Settings.XNum"=w546)  [unwired: 1 in, 2 out]
                    n174 = Subtract(x=w548, y=w544) -> (x-y=w547:dbl)
                    n175 = Quotient & Remainder(x=w547, y=w546) -> (floor(x/y)=w545:dbl)  [unwired: 1 out]
                    n176 = for {
                      N: w546 -> [_]
                      tunnel: w545 -> [w552]
                      tunnel: w544 -> [w550]
                      tunnel: [w549] -> w542 mode=indexing
                      i -> [w553]
                      n177 = Multiply(x=w552, y=w553) -> (x*y=w551:i32)
                      n178 = Add(x=w550, y=w551) -> (x+y=w549:i32)
                    }
                    "XPos" <- w542
                  }
                  frame #1 {
                    n179 = xnode "Read/Write Control"("FPGA VI Reference In"=w564) -> ("Scan Settings.YEnd"=w569, "Scan Settings.YStart"=w565, "Scan Settings.YNum"=w567)  [unwired: 1 in, 2 out]
                    n180 = Subtract(x=w569, y=w565) -> (x-y=w568:dbl)
                    n181 = Quotient & Remainder(x=w568, y=w567) -> (floor(x/y)=w566:dbl)  [unwired: 1 out]
                    n182 = for {
                      N: w567 -> [_]
                      tunnel: w566 -> [w573]
                      tunnel: w565 -> [w571]
                      tunnel: [w570] -> w563 mode=indexing
                      i -> [w574]
                      n183 = Multiply(x=w573, y=w574) -> (x*y=w572:i32)
                      n184 = Add(x=w571, y=w572) -> (x+y=w570:i32)
                    }
                    "YPos" <- w563
                  }
                  frame #2 {
                    n185 = xnode "Read/Write Control"("FPGA VI Reference In"=w590) -> ("Scan Settings.ZEnd"=w589, "Scan Settings.ZStart"=w585, "Scan Settings.ZNum"=w587)  [unwired: 1 in, 2 out]
                    n186 = Subtract(x=w589, y=w585) -> (x-y=w588:dbl)
                    n187 = Quotient & Remainder(x=w588, y=w587) -> (floor(x/y)=w586:dbl)  [unwired: 1 out]
                    n188 = for {
                      N: w587 -> [_]
                      tunnel: w586 -> [w594]
                      tunnel: w585 -> [w592]
                      tunnel: [w591] -> w584 mode=indexing
                      i -> [w595]
                      n189 = Multiply(x=w594, y=w595) -> (x*y=w593:i32)
                      n190 = Add(x=w592, y=w593) -> (x+y=w591:i32)
                    }
                    "ZPos" <- w584
                  }
                }
                n191 = local read "NumChans"() -> (w540:u32)
                n192 = xnode "Read/Write Control"("FPGA VI Reference In"=w539) -> ("Scan Settings.XNum"=w538, "Scan Settings.YNum"=w537, "Scan Settings.ZNum"=w536)  [unwired: 1 in, 2 out]
                n193 = for {
                  N: w536 -> [_]
                  tunnel: [w607] -> _ mode=indexing
                  tunnel: w540 -> [w605]
                  i -> [w606]
                  n194 = for {
                    N: w605 -> [_]
                    tunnel: [w613] -> w607 mode=indexing
                    tunnel: w606 -> [w612]
                    i -> [w611]
                    w608 = T14 0 items=["Grayscale (U8)", "Grayscale (I16)", "Grayscale (SGL)", "Complex (CSG)", "RGB (U32)", "HSL (U32)", "RGB (U64)", "Grayscale (U16)"] ("Image Type")
                    n195 = Format Into String(format string="%u_%u", w612, w611) -> (resulting string=w609:string)  [unwired: 2 in, 1 out]
                    n196 = call "IMAQ Create"("Image Name"=w609, "Image Type"=w608) -> ("New Image"=w613:T9)  [unwired: 3 in, 1 out]
                  }
                }
                n197 = local read "Scans"() -> (w535:i32)
                n198 = Compound Arithmetic op=MULTIPLY(w538, w537, w536, w535) -> (w534:i32)
                n199 = local write "Tab Control"(T3."Image Stack" ("Tab Control")) -> ()
              }
            }
            "TotalSamples" <- w517
            n200 = local read "StackSize"() -> (w522:cluster{"nX":u32, "nY":u32, "nZ":u32})
            n201 = Bundle By Name(cluster=w522, "nX"=w523, "nY"=w511, "nZ"=w524) -> (→"StackSize":cluster{"nX":u32, "nY":u32, "nZ":u32})
          }
          frame #1 {
            n202 = Or(x="SaveStream", y="SaveImage") -> (x .or. y?=w633:bool)
            n203 = case shown="True" w633 {
              tunnel: [w636 w641] -> w632
              frame #0 {
                (unwired) FALSE
                (unwired) u32 0 ("file handle")
                n204 = local read "StreamInfo"() -> (w638:T5)
                n205 = Bundle By Name(cluster=w638, "Open"=FALSE) -> (w636:T5)
              }
              frame #1 {
                w642 = "image" ("group name (empty)")
                n206 = local read "Mode"() -> (w644:enum16{"Points", "Volume", "Idle"})
                n207 = local read "NumChans"() -> (w639:u32)
                n208 = call <instrlib>:"niHWS Open File.vi"("permissions (0:read only)"=niHWS_Open_File_Permissions_ID."Read/Write/Create New", "file path"="Path") -> ("file handle"=w643:u32)  [unwired: 8 in, 1 out]
                n209 = local read "Scans"() -> (w640:i32)
                n210 = case shown="\"Volume\"" w644 {
                  tunnel: w643 -> [w666 w682]
                  tunnel: w642 -> [w665 w681]
                  tunnel: w640 -> [_ w667]
                  frame #0 {
                    n211 = local read "Points"() -> (w662:i32[][])
                    n212 = Array Size(array=w662) -> (size(s)=w663:i32[])
                    n213 = call <instrlib>:"niHWS New Wfm Reference.vi"("waveform name (empty)"="points", "group name (empty)"=w665, "file handle in"=w666) -> ("waveform reference"=w659:u32)  [unwired: 6 in, 2 out]
                    n214 = Multiply Array Elements(1:w663) -> (0:w661:i32)
                    n215 = Reshape Array(w662, w661) -> (w660:i32[])
                    n216 = call-poly <instrlib>:"niHWS Write.vi"("data"=w660, "waveform reference in"=w659) -> ()  [unwired: 8 in, 2 out]
                  }
                  frame #1 {
                    n217 = local read "Scan Settings"() -> (w680:T4)
                    n218 = call <instrlib>:"niHWS New Wfm Reference.vi"("waveform name (empty)"="volume_settings", "group name (empty)"=w681, "file handle in"=w682) -> ("waveform reference"=w670:u32)  [unwired: 6 in, 2 out]
                    n219 = Unbundle By Name(w680) -> ("XStart"=w679:i32, "XEnd"=w678:i32, "XNum"=w677:i32, "YStart"=w676:i32, "YEnd"=w675:i32, "YNum"=w674:i32, "ZStart"=w673:i32, "ZEnd"=w672:i32, "ZNum"=w668:i32)
                    n220 = Build Array(w679, w678, w677, w676, w675, w674, w673, w672, w668, w667) -> (w671:i32[])
                    n221 = call-poly <instrlib>:"niHWS Write.vi"("data"=w671, "waveform reference in"=w670) -> ()  [unwired: 8 in, 2 out]
                  }
                }
                n222 = call <instrlib>:"niHWS New Wfm Reference.vi"("waveform name (empty)"="stream", "group name (empty)"="stream", "file handle in"=w643) -> ("waveform reference"=w651:u32, "file handle out"=w648:u32)  [unwired: 6 in, 1 out]
                n223 = Build Array(w644, w639) -> (w646:u32[])
                n224 = call <instrlib>:"niHWS New Wfm Reference.vi"("waveform name (empty)"="Mode", "group name (empty)"=w642, "file handle in"=w643) -> ("waveform reference"=w645:u32)  [unwired: 6 in, 2 out]
                n225 = call <instrlib>:"niHWS New Wfm Reference.vi"("waveform name (empty)"="image", "group name (empty)"=w642, "file handle in"=w648) -> ("waveform reference"=w652:u32, "file handle out"=w649:u32)  [unwired: 6 in, 1 out]
                n226 = call-poly <instrlib>:"niHWS Write.vi"("data"=w646, "waveform reference in"=w645) -> ()  [unwired: 8 in, 2 out]
                n227 = local read "StreamInfo"() -> (w653:T5)
                n228 = Bundle By Name(cluster=w653, "Open"=TRUE, "file handle out"=w649, "image reference"=w652, "stream reference"=w651) -> (w641:T5)
              }
            }
            "StreamInfo" <- w632
          }
          frame #2 {
            n229 = local read "FPGA VI Execution Mode"() -> (w688:T6)
            n230 = case shown="\"FPGA Target\", Default" w688 {
              tunnel: w687 -> [w705 _]
              tunnel: w686 -> [w694 w825]
              tunnel: w685 -> [w693 w824]
              tunnel: [w692 w824] -> w684
              tunnel: [w691 w825] -> w683
              frame #0 {
                n231 = flat-sequence {
                  tunnel: w705 -> [w716]
                  tunnel: [w715] -> w714
                  tunnel: w714 -> [w731]
                  tunnel: [w729] -> w697
                  tunnel: [w752] -> w704
                  tunnel: [w755] -> w701
                  tunnel: [w754] -> w699
                  tunnel: w697 -> [w753]
                  tunnel: [w753] -> w696
                  tunnel: [w751] -> w695
                  tunnel: w704 -> [w768]
                  tunnel: [w768] -> w703
                  tunnel: [w767] -> w702
                  tunnel: w701 -> [w766]
                  tunnel: [w766] -> w700
                  tunnel: w699 -> [w765]
                  tunnel: [w765] -> w698
                  tunnel: w696 -> [w764]
                  tunnel: w695 -> [w767]
                  tunnel: w694 -> [w762]
                  tunnel: w693 -> [w761]
                  tunnel: [w760] -> w692
                  tunnel: [w759] -> w691
                  tunnel: [w757] -> w689
                  tunnel: w703 -> [w789]
                  tunnel: [w787] -> w713
                  tunnel: w702 -> [w786]
                  tunnel: [w785] -> w712
                  tunnel: [w784] -> w711
                  tunnel: w700 -> [w784]
                  tunnel: w698 -> [w783]
                  tunnel: [w783] -> w710
                  tunnel: [w782] -> w690
                  tunnel: w689 -> [w782]
                  tunnel: w713 -> [w798]
                  tunnel: w712 -> [w797]
                  tunnel: [w796] -> w709
                  tunnel: [w795] -> w708
                  tunnel: [w793] -> w707
                  tunnel: w711 -> [w793]
                  tunnel: [w792] -> w706
                  tunnel: w710 -> [w792]
                  tunnel: w690 -> [w791]
                  tunnel: w709 -> [w823]
                  tunnel: w708 -> [w822]
                  tunnel: w707 -> [w821]
                  tunnel: w706 -> [w820]
                  frame #0 {
                    n232 = while {
                      tunnel: w716 -> [w719]
                      tunnel: [w717] -> w715
                      stop <- w718 stop-if-true
                      n233 = xnode "Read/Write Control"("FPGA VI Reference In"=w719) -> ("FPGA VI Reference Out"=w717:T10, "Armed"=w718)  [unwired: 1 in, 1 out]
                    }
                  }
                  frame #1 {
                    n234 = xnode "Read/Write Control"("FPGA VI Reference In"=w731, "ExtAcqTrig"=FALSE) -> ("FPGA VI Reference Out"=w729:T10)  [unwired: 1 in, 1 out]
                    n235 = Wait (ms)(milliseconds to wait=u32 50) -> ()  [unwired: 1 out]
                  }
                  frame #2 {
                    w754 = tag "/PXI1Slot5/PXI_Trig0" ("destination terminal")
                    w755 = tag "/PXI1Slot5/PFI0" ("source terminal")
                    n236 = call-poly <vilib>:"DAQmx Create Virtual Channel.vi"("lines"=tag "PXI1Slot5/port0/line0") -> ("task out"=w750:refnum<k21>, "error out"=w749:errorcluster)  [unwired: 13 in]
                    n237 = Wait (ms)(milliseconds to wait=u32 100) -> ()  [unwired: 1 out]
                    n238 = call-poly <vilib>:"DAQmx Write.vi"("task/channels in"=w750, "auto start"=TRUE, "data"=FALSE, "error in"=w749) -> ("task out"=w752:refnum<k21>, "error out"=w751:errorcluster)  [unwired: 9 in, 1 out]
                    n239 = call <vilib>:"DAQmx Connect Terminals.vi"("source terminal"=w755, "destination terminal"=w754) -> ()  [unwired: 13 in, 1 out]
                  }
                  frame #3 {
                    n240 = xnode "Read/Write Control"("FPGA VI Reference In"=w764, "ExtAcqTrig"=TRUE) -> ("FPGA VI Reference Out"=w757:T10)  [unwired: 1 in, 1 out]
                    n241 = call <vilib>:"DAQmx Start Task.vi"("task/channels in"=w762, "error in"=w761) -> ("task out"=w759:refnum<k21>, "error out"=w760:errorcluster)  [unwired: 12 in]
                    n242 = Wait (ms)(milliseconds to wait=u32 100) -> ()  [unwired: 1 out]
                  }
                  frame #4 {
                    n243 = call-poly <vilib>:"DAQmx Write.vi"("task/channels in"=w789, "data"=TRUE, "error in"=w786) -> ("task out"=w787:refnum<k21>, "error out"=w785:errorcluster)  [unwired: 10 in, 1 out]
                  }
                  frame #5 {
                    w790 = FALSE ("ExtAcqTrig")
                    n244 = xnode "Read/Write Control"("FPGA VI Reference In"=w791, "ExtAcqTrig"=w790, "TriggerAcq"=w790, "Volume Scan"=w790) -> ()  [unwired: 1 in, 2 out]
                    n245 = call-poly <vilib>:"DAQmx Write.vi"("task/channels in"=w798, "data"=FALSE, "error in"=w797) -> ("task out"=w796:refnum<k21>, "error out"=w795:errorcluster)  [unwired: 10 in, 1 out]
                  }
                  frame #6 {
                    n246 = call <vilib>:"DAQmx Disconnect Terminals.vi"("source terminal"=w821, "destination terminal"=w820) -> ()  [unwired: 13 in, 1 out]
                    n247 = call <vilib>:"DAQmx Clear Task.vi"("task in"=w823, "error in"=w822) -> ()  [unwired: 13 in, 1 out]
                  }
                }
              }
              frame #1 {
              }
            }
          }
        }
      }
      frame #3 {
        # "Take data and shuffle between various FIFO's and queues\n(producer loop)"
        n248 = local read "TotalSamples"() -> (w862:u32)
        n249 = local read "Downsample"() -> (w858:i32)
        n250 = local read "PMT Read"() -> (w847:i32)
        n251 = local read "ImCh Read"() -> (w845:i32)
        n252 = Subtract(x=w862, y=w845) -> (x-y=w861:u32)
        n253 = Multiply(x="ImReadSize", y=w858) -> (x*y=w837:i32)
        n254 = Multiply(x=w858, y=w862) -> (x*y=w859:u32)
        n255 = To Unsigned Long Integer(number=w847) -> (unsigned 32bit integer=w857:u32)
        n256 = Greater Than 0?(x=w861) -> (x > 0?=w849:bool)
        n257 = local read "FPGA VI Execution Mode"() -> (w846:T6)
        n258 = Not(x="Abort") -> (.not. x?=w848:bool)
        n259 = Subtract(x=w859, y=w857) -> (x-y=w836:u32)
        n260 = And(x=w848, y=w849) -> (x .and. y?=w850:bool)
        n261 = Max & Min(x=w837, y=w836) -> (min(x,y)=w835:u32)  [unwired: 1 out]
        n262 = local read "PMT Read"() -> (w830:i32)
        n263 = xnode "Read/Write Control"("FPGA VI Reference In"=w839, "Abort"="Abort") -> ()  [unwired: 1 in, 2 out]
        n264 = Select(t=u32 0, s="Abort", f=w835) -> (s? t:f=w851:u32)
        n265 = Equal To 0?(x=w830) -> (x = 0?=w829:bool)
        n266 = local read "NumChans"() -> (w831:u32)
        n267 = Select(t=w828, s=w829, f=0.0) -> (s? t:f=w826:dbl)
        n268 = case shown="True" w850 {
          tunnel: w839 -> [_ w969]
          tunnel: w845 -> [_ _]
          tunnel: "ImReadSize" -> [_ w970]
          tunnel: [TRUE FALSE] -> w843
          tunnel: w861 -> [_ w971]
          tunnel: w845 -> [_ w958]
          frame #0 {
          }
          frame #1 {
            n269 = local read "NumChans"() -> (w964:u32)
            n270 = Max & Min(x=w970, y=w971) -> (min(x,y)=w968:u32)  [unwired: 1 out]
            n271 = Multiply(x=w964, y=w968) -> (x*y=w967:u32)
            n272 = xnode "Invoke Method"("FPGA VI Reference In"=w969, "Number of Elements"=w967, "Timeout (ms)"=5) -> ("error out"=w961:errorcluster, "Data"=w956:i32[], "Elements Remaining"=→"ImCh Backlog":u32)  [unwired: 1 in, 1 out]
            n273 = Array Size(array=w956) -> (size(s)=w965:i32)
            n274 = call <vilib>:"Clear Errors.vi"("error in (no error)"=w961) -> ()  [unwired: 6 in, 1 out]
            n275 = Divide(x=w965, y=w964) -> (x/y=w962:dbl)
            n276 = local read "voxel queue"() -> (w957:refnum<queue>)
            n277 = To Unsigned Long Integer(number=w962) -> (unsigned 32bit integer=w963:u32)
            n278 = Add(x=w963, y=w958) -> (x+y=→"ImCh Read":u32)
            n279 = Enqueue Element(queue=w957, element=w956) -> ()  [unwired: 2 in, 3 out]
          }
        }
        n280 = Multiply(x=w831, y=w826) -> (x*y=w834:dbl)
        n281 = Divide(x=w834, y=2 ("x")) -> (x/y=w833:dbl)
        n282 = case shown="1, Default" w851 {
          selector: w851 -> [_ w912]
          tunnel: [w882 w924] -> w867
          tunnel: w854 -> [w883 w921]
          tunnel: w853 -> [w885 w923]
          tunnel: [w884 w922] -> w855
          tunnel: w839 -> [_ w918]
          tunnel: w846 -> [_ w915]
          tunnel: [TRUE FALSE] -> w840
          tunnel: w826 -> [_ w910]
          tunnel: w833 -> [_ w908]
          frame #0 {
            n283 = local read "FPGA VI Execution Mode"() -> (w886:T6)
            n284 = case shown="\"FPGA Target\", Default" w886 {
              tunnel: w885 -> [w892 w901]
              tunnel: [w888 w901] -> w884
              tunnel: [w887 w900] -> w882
              tunnel: w883 -> [w893 w900]
              frame #0 {
                n285 = property class="DAQmx Task"(reference=w893, error in=w892) -> (reference out=w890:refnum<k21>, error out=w889:errorcluster, "Done"=w891:bool)
                n286 = case shown="True" w891 {
                  tunnel: w890 -> [w897 w898]
                  tunnel: w889 -> [w896 w899]
                  tunnel: [w895 w899] -> w888
                  tunnel: [w894 w898] -> w887
                  frame #0 {
                    n287 = call <vilib>:"DAQmx Stop Task.vi"("task/channels in"=w897, "error in"=w896) -> ("task out"=w894:refnum<k21>, "error out"=w895:errorcluster)  [unwired: 12 in]
                  }
                  frame #1 {
                  }
                }
              }
              frame #1 {
              }
            }
          }
          frame #1 {
            n288 = Add(x=w910, y=w912) -> (x+y=w911:dbl)
            n289 = case shown="\"FPGA Target\", Default" w915 {
              tunnel: [w945 w954] -> w924
              tunnel: w923 -> [w944 w953]
              tunnel: [w942 w951] -> w909
              tunnel: w911 -> [w941 w950]
              tunnel: [w940 w953] -> w922
              tunnel: w921 -> [w938 w954]
              frame #0 {
                n290 = property class="DAQmx Read"(reference=w938) -> ("AvailSampPerChan"=→"PMT Backlog":u32)  [unwired: 1 in, 2 out]
                n291 = call-poly <vilib>:"DAQmx Read.vi"("task/channels in"=w938, "number of samples per channel"=w941, "timeout"=2.0, "error in"=w944) -> ("task out"=w945:refnum<k21>, "data"=w942:i32[], "error out"=w940:errorcluster)  [unwired: 9 in]
              }
              frame #1 {
                n292 = local read "NumChans"() -> (w947:u32)
                n293 = Divide(x=w950, y=u32 2) -> (x/y=w948:dbl)
                n294 = Divide(x=w948, y=w947) -> (x/y=w946:dbl)
                n295 = call <vilib>:"Ramp Pattern.vi"("samples"=w946) -> ("Ramp Pattern"=w952:dbl[])  [unwired: 9 in, 1 out]
                n296 = To Unsigned Long Integer(number=w952) -> (unsigned 32bit integer=w951:u32[])
              }
            }
            n297 = Split 1D Array(array=w909, index=w908) -> (second subarray=w907:u32[])  [unwired: 1 out]
            n298 = xnode "Invoke Method"("FPGA VI Reference In"=w918, "Data"=w907, "Timeout (ms)"=-1) -> ("Empty Elements Remaining"=→"PMT FIFO Space":u32)  [unwired: 1 in, 2 out]
            n299 = local read "NumChans"() -> (w906:u32)
            n300 = Array Size(array=w907) -> (size(s)=w917:i32)
            n301 = Multiply(x=w917, y=2) -> (x*y=w905:i32)
            n302 = Divide(x=w905, y=w906) -> (x/y=w904:dbl)
            n303 = local read "SaveStream"() -> (w914:bool)
            n304 = local read "PMT Read"() -> (w902:i32)
            n305 = Add(x=w902, y=w904) -> (x+y=→"PMT Read":dbl)
            n306 = case shown="True" w914 {
              tunnel: w907 -> [_ w926]
              frame #0 {
              }
              frame #1 {
                n307 = local read "raw out"() -> (w925:refnum<queue>)
                n308 = Enqueue Element(queue=w925, element=w926) -> ()  [unwired: 2 in, 3 out]
              }
            }
          }
        }
        n309 = local read "Abort"() -> (w842:bool)
        n310 = And(x=w840, y=w843) -> (x .and. y?=w841:bool)
        n311 = Unbundle By Name(w855) -> ("status"=w856:bool)
        n312 = Compound Arithmetic op=OR(w856, w841, w842) -> (w860:bool)
        n313 = Select(t=T2."End Acquire", s=w860, f=T2."Acquire") -> (s? t:f=w866:T2)
        "Throwaway Samples" <- w828
      }
      frame #4 {
        w1003 = T15 2 items=["no dialog", "OK message", "continue or stop message", "OK message + warnings", "continue/stop + warnings"] ("type of dialog (OK msg:1)")
        n314 = local read "Processing"() -> (w991:bool)
        n315 = xnode "Read/Write Control"("FPGA VI Reference In"=w1001, "TriggerAcq"=FALSE) -> ()  [unwired: 1 in, 2 out]
        n316 = Not(x=w991) -> (.not. x?=w992:bool)
        n317 = call <vilib>:"General Error Handler.vi"("type of dialog (OK msg:1)"=w1003, "error in (no error)"=w1004) -> ("error out"=w999:errorcluster)  [unwired: 9 in, 4 out]
        n318 = feedback #5() -> (w993:bool)  [unwired: 1 in]
        n319 = feedback #6() -> (w994:bool)  [unwired: 1 in]
        n320 = Not(x=w991) -> (.not. x?=w996:bool)
        n321 = feedback #7() -> (w995:bool)  [unwired: 1 in]
        n322 = Compound Arithmetic op=AND(w992, w993, w994) -> (w989:bool)
        n323 = And(x=w996, y=w995) -> (x .and. y?=w990:bool)
        n324 = Or(x=w990, y=w989) -> (x .or. y?=w988:bool)
        n325 = case shown="True" w988 {
          tunnel: [T2."Reset" T2."End Acquire"] -> w997
          frame #0 {
            n326 = local read "StreamInfo"() -> (w1007:T5)
            n327 = Bundle By Name(cluster=w1007, "Open"=FALSE) -> (w1009:T5)
            n328 = Unbundle By Name(w1007) -> ("file handle out"=w1010:u32, "Open"=w1005:bool)
            n329 = local write "StreamInfo"(w1009) -> ()
            n330 = case shown="True" w1005 {
              tunnel: w1010 -> [_ w1011]
              frame #0 {
              }
              frame #1 {
                n331 = call <instrlib>:"niHWS Close File.vi"("file handle"=w1011) -> ()  [unwired: 10 in, 1 out]
              }
            }
          }
          frame #1 {
            n332 = Wait (ms)(milliseconds to wait=u32 50) -> ()  [unwired: 1 out]
          }
        }
      }
    }
    "Loop Count" <- w195
    "Host State" <- w190
  }
  n333 = while {
    shift-right: [w1029] -> _
    shift-left: _ -> [w1028]
    shift-right: [w1031] -> _
    shift-left: _ -> [w1032]
    stop <- w1027 stop-if-true
    n334 = event shown="[1] \"Section\": Value Change" {
      selector: _ -> [_ _ _ _ _]
      dyn-events: _ -> [_ _ _ _ _]
      timeout: 500 -> [_ _ _ _ _]
      tunnel: w1032 -> [w1045 w1061 w1079 w1121 w1129]
      tunnel: [w1046 w1061 w1072 w1120 w1128] -> w1031
      tunnel: [w1036 w1059 w1073 w1119 w1133] -> w1029
      tunnel: w1028 -> [w1036 w1059 w1073 w1119 w1131]
      event #0 {
        n335 = event-data() -> ()  [unwired: 1 in, 2 out]
        n336 = local read "Host State"() -> (w1043:T2)
        n337 = property on="ImCh1 2" class="ImageControl"() -> ("ROI"=w1044:T16)  [unwired: 2 in, 2 out]
        n338 = local read "Mode"() -> (w1041:enum16{"Points", "Volume", "Idle"})
        n339 = Equal?(x=enum16{"Points", "Volume", "Idle"}."Volume", y=w1041) -> (x = y?=w1039:bool)
        n340 = Not Equal?(x=w1043, y=T2."Idle") -> (x != y?=w1038:bool)
        n341 = Replace Array Subset(array=w1045, new element=w1044) -> (w1046:T17)  [unwired: 1 in]
        n342 = And(x=w1038, y=w1039) -> (x .and. y?=w1037:bool)
        n343 = Divide(x="Max", y=255.0) -> (x/y=w1033:dbl)
        n344 = case shown="True" w1037 {
          tunnel: w1036 -> [_ w1049]
          tunnel: w1033 -> [_ w1047]
          frame #0 {
          }
          frame #1 {
            n345 = local read "ImData"() -> (w1048:i32[][])
            n346 = local read "ImCh1 2"() -> (w1054:T9)
            n347 = local read "ImCh2 2"() -> (w1053:T9)
            n348 = Divide(x=w1048, y=w1047) -> ()  [unwired: 1 out]
            n349 = call "UpdateStack.vi"("Scan Settings"=w1049, "Section"="Section", "ImData"=w1048, "Im2 2"=w1053, "Im1 In"=w1054) -> ("Im2 Out"=→"ImCh2 2":T9, "Im1 Out"=→"ImCh1 2":T9)  [unwired: 5 in]
          }
        }
      }
      event #1 {
        n350 = event-data() -> ("NewVal"=w1060:i32)  [unwired: 1 in, 4 out]
        n351 = local read "Max"() -> (w1056:u32)
        n352 = Divide(x=w1056, y=u8 255) -> (x/y=w1057:dbl)
        n353 = local read "Display Data"() -> (w1058:bool)
        n354 = case shown="True" w1058 {
          tunnel: w1060 -> [_ w1067]
          tunnel: w1059 -> [_ w1066]
          tunnel: w1057 -> [_ w1063]
          frame #0 {
          }
          frame #1 {
            n355 = local read "ImData"() -> (w1065:i32[][])
            n356 = local read "ImCh1 2"() -> (w1070:T9)
            n357 = local read "ImCh2 2"() -> (w1071:T9)
            n358 = Divide(x=w1065, y=w1063) -> (x/y=w1064:dbl[][])
            n359 = call "UpdateStack.vi"("Scan Settings"=w1066, "Section"=w1067, "ImData"=w1064, "Im2 2"=w1071, "Im1 In"=w1070) -> ("Im2 Out"=w1069:T9, "Im1 Out"=w1068:T9)  [unwired: 5 in]
            n360 = local write "ImCh2 2"(w1069) -> ()
            n361 = local write "ImCh1 2"(w1068) -> ()
          }
        }
        n362 = Index Array(array=w1061, index=w1060) -> (element=w1062:T16)
        n363 = property on="ImCh1 2" class="ImageControl"("ROI"=w1062) -> ()  [unwired: 2 in, 2 out]
      }
      event #2 {
        n364 = event-data() -> ()  [unwired: 1 in, 7 out]
        n365 = local read "Section"() -> (w1077:i32)
        n366 = property on="ImCh1 2" class="ImageControl"() -> ("ROI"=w1078:T16)  [unwired: 2 in, 2 out]
        n367 = Replace Array Subset(array=w1079, new element=w1078, index=w1077) -> (w1072:T17)
        n368 = for {
          tunnel: w1072 -> [w1086] mode=indexing
          shift-right: [w1082] -> w1076
          shift-left: i32[][] [] -> [w1083]
          tunnel: w1073 -> [w1081]
          tunnel: "GridPoints" -> [w1080]
          i -> [w1084]
          n369 = Unbundle By Name(w1086) -> ("Contours"=w1085:T18)
          n370 = for {
            tunnel: w1085 -> [w1094] mode=indexing
            tunnel: w1084 -> [w1090]
            shift-right: [w1089] -> w1082
            shift-left: w1083 -> [w1091]
            tunnel: w1081 -> [w1088]
            tunnel: w1080 -> [w1087]
            n371 = Unbundle By Name(w1094) -> ("ROI Type"=w1093:u32, "Points"=w1092:i32[])
            n372 = case shown="1" w1093 {
              tunnel: w1092 -> [_ w1102 w1110 w1115]
              tunnel: w1091 -> [w1095 w1100 w1106 w1118]
              tunnel: w1090 -> [_ w1101 w1109 w1117]
              tunnel: [w1095 w1099 w1104 w1116] -> w1089
              tunnel: w1088 -> [_ w1097 w1108 w1114]
              tunnel: w1087 -> [_ _ w1103 w1111]
              frame #0 {
              }
              frame #1 {
                n373 = Build Array (concatenate)(w1102, w1101) -> (w1096:i32[])
                n374 = call "PointToSetting.vi"("Clicked"=w1096, "Scan Settings"=w1097) -> ("Setting"=w1098:i32[])  [unwired: 9 in]
                n375 = Build Array (concatenate)(w1100, w1098) -> (w1099:i32[][])
              }
              frame #2 {
                n376 = Build Array (concatenate)(w1110, w1109) -> (w1107:i32[])
                n377 = call "LineToSetting.vi"("GridSize"=w1103, "Line"=w1107, "Scan Settings"=w1108) -> ("Settings"=w1105:i32[][])  [unwired: 8 in]
                n378 = Build Array (concatenate)(w1106, w1105) -> (w1104:i32[][])
              }
              frame #3 {
                n379 = Build Array (concatenate)(w1115, w1117) -> (w1112:i32[])
                n380 = call "BoxToSetting.vi"("GridSize"=w1111, "Line"=w1112, "Scan Settings"=w1114) -> ("Settings"=w1113:i32[][])  [unwired: 8 in]
                n381 = Build Array (concatenate)(w1118, w1113) -> (w1116:i32[][])
              }
            }
          }
        }
        n382 = local write "Points"(w1076) -> ()
      }
      event #3 {
        n383 = event-data() -> ("NewVal"=w1122:bool)  [unwired: 1 in, 4 out]
        n384 = case shown="True" w1122 {
          tunnel: w1121 -> [w1123 _]
          tunnel: [w1123 w1127] -> w1120
          tunnel: w1119 -> [_ w1125]
          frame #0 {
          }
          frame #1 {
            w1126 = T16 {"Global Rectangle"=[], "Contours"=[]} ("ROI")
            n385 = Unbundle By Name(w1125) -> ("ZNum"=w1124:i32)
            n386 = Initialize Array(w1126, w1124) -> (w1127:T17)
            n387 = property on="ImCh1 2" class="ImageControl"("ROI"=w1126) -> ()  [unwired: 2 in, 2 out]
          }
        }
      }
      event #4 {
        n388 = event-data() -> ()  [unwired: 1 in, 5 out]
        n389 = local read "Scan Settings"() -> (w1132:T4)
        n390 = Equal?(x=w1132, y=w1131) -> (x = y?=w1130:bool)
        n391 = case shown="False" w1130 {
          tunnel: w1132 -> [w1136 w1139]
          tunnel: [w1136 w1139] -> w1133
          tunnel: [w1135 w1138] -> w1128
          tunnel: w1129 -> [_ w1138]
          frame #0 {
            w1137 = T16 {"Global Rectangle"=[], "Contours"=[]} ("ROI")
            n392 = Unbundle By Name(w1136) -> ("ZNum"=w1134:i32)  [unwired: 2 out]
            n393 = property on="Section" class="Scroll (strict)"("DocMax"=w1134) -> ()  [unwired: 2 in, 2 out]
            n394 = Initialize Array(w1137, w1134) -> (w1135:T17)
            n395 = property on="ImCh1 2" class="ImageControl"("ROI"=w1137) -> ()  [unwired: 2 in, 2 out]
          }
          frame #1 {
          }
        }
      }
    }
    n396 = local read "Stop"() -> (w1027:bool)
  }
  n397 = case shown="\"FPGA Target\", Default" w19 {
    tunnel: [w1140 w1150] -> w32
    tunnel: w30 -> [w1141 w1150]
    frame #0 {
      w1142 = T11 5 items=["PXI_Trig0", "PXI_Trig1", "PXI_Trig2", "PXI_Trig3", "PXI_Trig4", "PXI_Trig5", "PXI_Trig6", "PXI_Trig7"] ("Trigger")
      n398 = xnode "Invoke Method"("FPGA VI Reference In"=w1141, "Trigger"=w1142) -> ("FPGA VI Reference Out"=w1140:T10)  [unwired: 1 in, 1 out]
    }
    frame #1 {
    }
  }
  n399 = call <vilib>:"DAQmx Stop Task.vi"("task/channels in"=w28, "error in"=w27) -> ()  [unwired: 12 in, 2 out]
  n400 = xnode "Close FPGA VI Reference"("FPGA VI Reference In"=w32) -> ()  [unwired: 1 in, 1 out]
